vi "Convert I64 to U32 with error if overflow.vi"(3 "error in":errorcluster, 5 "I64":i64) -> (0 "error out":errorcluster, 1 "Out of range?":bool, 2 "U32":u32)   [LabVIEW 2015, in "Tiff reader.lvlib"]
doc: "Converts I64 to U32, and returns an error if overflow."
uses:
  Tiff reader.lvlib
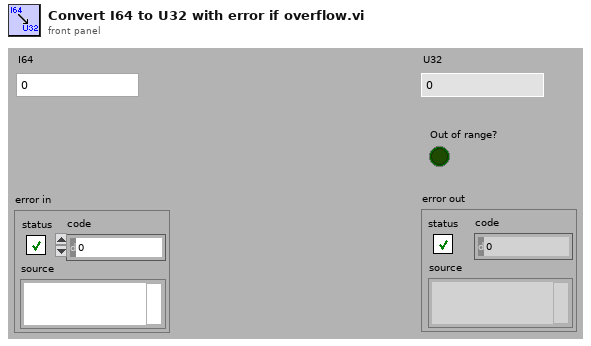
[diagram p1: front panel]
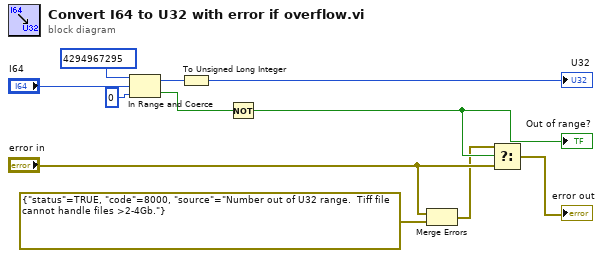
[diagram p0: block diagram]
diagram:
  n1 = In Range and Coerce(upper limit=i64 4294967295 ("dimension size"), x="I64", lower limit=i64 0) -> (coerced(x)=w8:i64, In Range?=w6:bool)
  n2 = To Unsigned Long Integer(number=w8) -> (unsigned 32bit integer=→"U32":u32)
  n3 = Not(x=w6) -> (.not. x?=w5:bool)
  "Out of range?" <- w5
  n4 = Merge Errors("error in", errorcluster {"status"=TRUE, "code"=8000, "source"="Number out of U32 range.  Tiff file cannot handle files >2-4Gb."} ("error out")) -> (w1:errorcluster)
  n5 = Select(t=w1, s=w5, f="error in") -> (s? t:f=→"error out":errorcluster)
